vi "Check&RPN.vi"(8 "error in (no error)":errorcluster, 11 "Array STEP":refnum<class "STEP.lvclass">[](array[class])) -> (0 "error out":errorcluster, 3 "STEP Out":refnum<class "STEP.lvclass">[](array[class]))   [LabVIEW 2014, in "SeqLoop.lvlib"]
uses:
  SeqLoop.lvlib
  Classes/STEP/STEP.lvclass
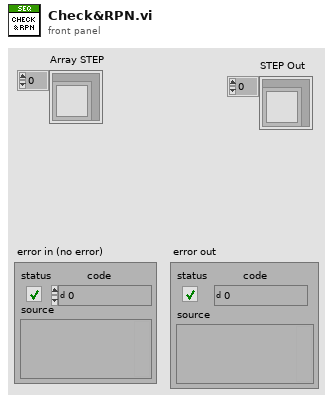
[diagram p1: front panel]
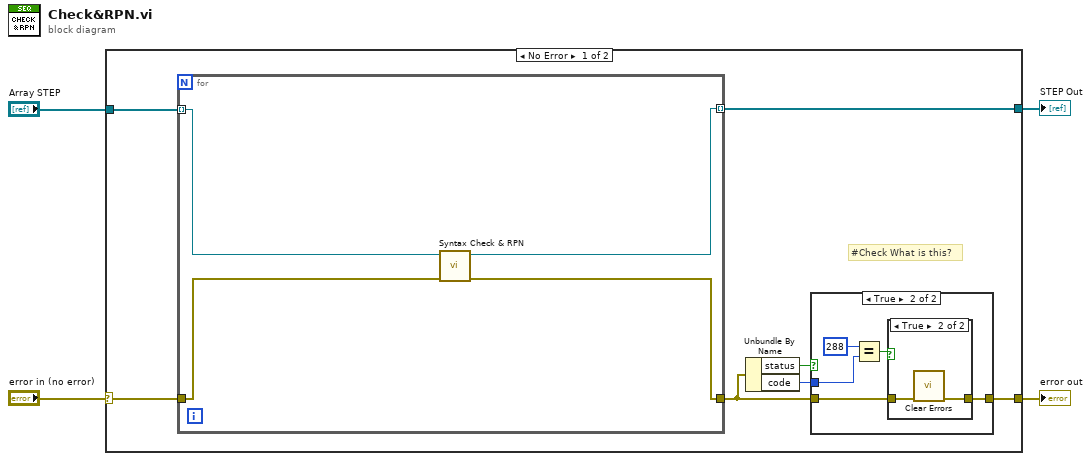
[diagram p0: block diagram]
diagram:
  n1 = case shown="No Error" "error in (no error)" {
    selector: "error in (no error)" -> [w5 w26]
    tunnel: [w8 w26] -> w3
    tunnel: "Array STEP" -> [w6 w25]
    tunnel: [w11 w25] -> w1
    frame No Error {
      # "#Check What is this?"
      n2 = for {
        tunnel: w5 -> [w24]
        tunnel: [w23] -> w7
        tunnel: w6 -> [w22] mode=indexing
        tunnel: [w21] -> w11 mode=indexing
        n3 = call "Syntax Check & RPN.vi"("error in (no error)"=w24, "STEP in"=w22) -> ("error out"=w23:errorcluster, "STEP out"=w21:refnum<class "STEP.lvclass">)  [unwired: 8 in]
      }
      n4 = Unbundle By Name(w7) -> ("status"=w9:bool, "code"=w10:i32)
      n5 = case shown="True" w9 {
        tunnel: [w12 w13] -> w8
        tunnel: w7 -> [w12 w14]
        tunnel: w10 -> [_ w17]
        frame False {
        }
        frame True {
          n6 = Equal?(x=288, y=w17) -> (x = y?=w15:bool)
          n7 = case shown="True" w15 {
            tunnel: w14 -> [w18 w20]
            tunnel: [w18 w19] -> w13
            frame False {
            }
            frame True {
              n8 = call <vilib>:"Clear Errors.vi"("error in (no error)"=w20) -> ("error out"=w19:errorcluster)  [unwired: 5 in, 1 out]
            }
          }
        }
      }
    }
    frame Error {
    }
  }
  "error out" <- w3
  "STEP Out" <- w1
